vi "Remove Repeated Correction Values (SubVI).vi"(11 "Compensation Out (%)":cluster{"xi used":dbl[], "yi":dbl[]}) -> (3 "Cluster":cluster{dbl[], dbl[]})   [LabVIEW 2016]
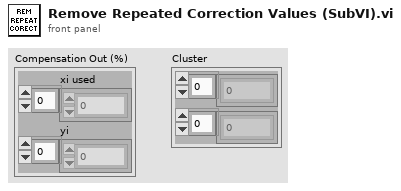
[diagram p1: front panel]
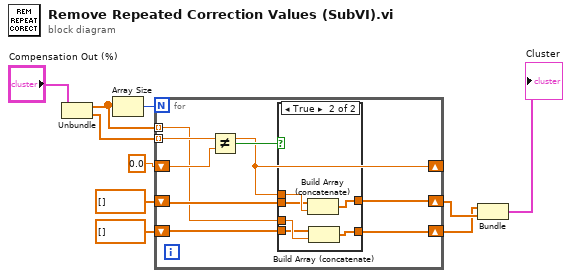
[diagram p0: block diagram]
diagram:
  n1 = Unbundle("Compensation Out (%)") -> ("xi used"=w4:dbl[], "yi"=w3:dbl[])
  n2 = Array Size(array=w4) -> (size(s)=w2:i32)
  n3 = for {
    N: w2 -> [_]
    tunnel: w3 -> [w16] mode=indexing
    tunnel: w4 -> [w13] mode=indexing
    shift-right: [w16] -> _
    shift-left: 0.0 ("Numeric") -> [w18]
    shift-right: [w14] -> w9
    shift-left: dbl[] [] -> [w15]
    shift-right: [w12] -> w8
    shift-left: dbl[] [] -> [w11]
    n4 = Not Equal?(x=w16, y=w18) -> (x != y?=w17:bool)
    n5 = case shown="True" w17 {
      tunnel: w16 -> [_ w24]
      tunnel: w15 -> [w20 w23]
      tunnel: [w20 w26] -> w14
      tunnel: w13 -> [_ w22]
      tunnel: [w19 w25] -> w12
      tunnel: w11 -> [w19 w21]
      frame False {
      }
      frame True {
        n6 = Build Array (concatenate)(w23, w24) -> (w26:dbl[])
        n7 = Build Array (concatenate)(w21, w22) -> (w25:dbl[])
      }
    }
  }
  n8 = Bundle(w8, w9) -> (→"Cluster":cluster{dbl[], dbl[]})  [unwired: 1 in]
